vi "linear_system.vi"(4 "c(friction)":dbl, 5 "k(spring force)":dbl, 6 "delta_t":dbl, 7 "m(mass)":dbl, 8 "u_in(input force)":dbl, 9 "a_init":dbl, 10 "v_init":dbl, 11 "x_init":dbl) -> (1 "a_out":dbl, 2 "v_out":dbl, 3 "x_out":dbl)   [LabVIEW 2019]
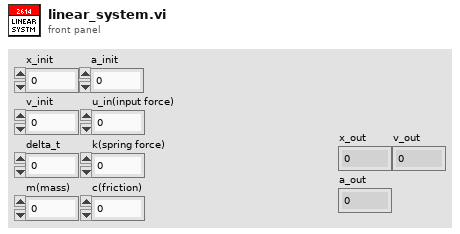
[diagram p1: front panel]
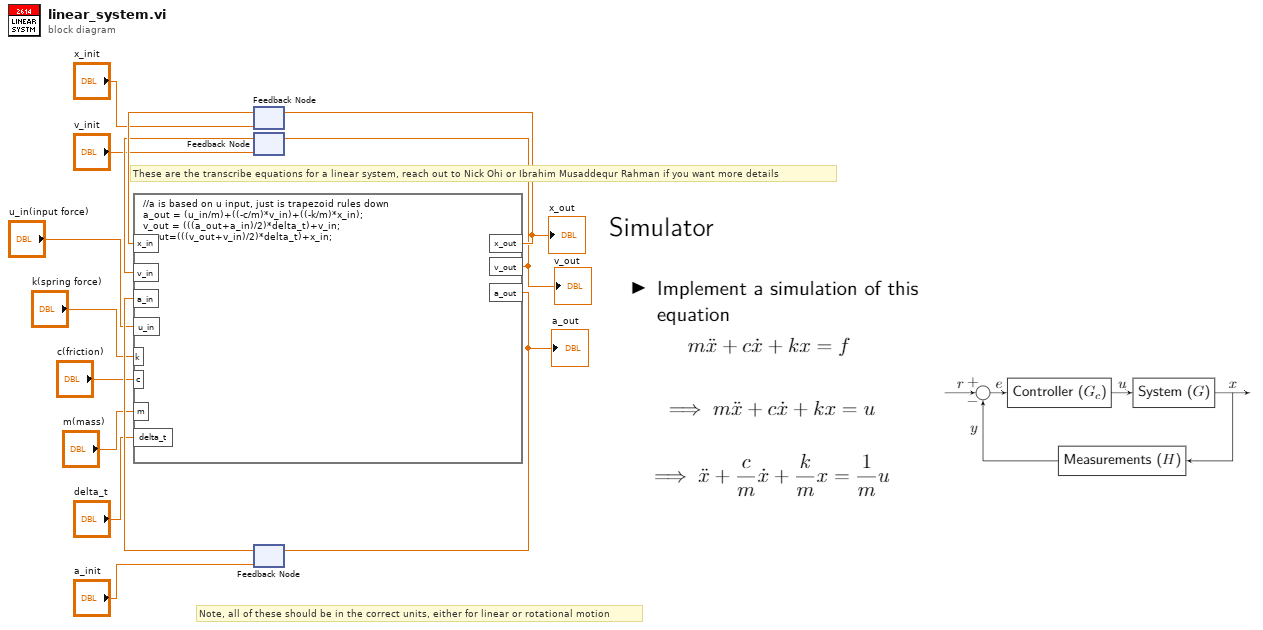
[diagram p0: block diagram]
diagram:
  # "These are the transcribe equations for a linear system, reach out to Nick Ohi or Ibrahim Musaddequr Rahman if you want more details"
  # "Note, all of these should be in the correct units, either for linear or rotational motion"
  n1 = feedback #1("x_init") -> (w14:dbl)
  n2 = feedback #2("v_init") -> (w10:dbl)
  n3 = feedback #3("a_init") -> (w7:dbl)
  n4 = formula code="//a is based on u input, just is trapezoid rules down\na_out = (u_in/m)+((-c/m)*v_in)+((-k/m)*x_in);\nv_out = (((a_out+a_in)/2)*delta_t)+v_in;\nx_out=(((v_out+v_in)/2)*delta_t)+x_in;"("x_in"=w14, "v_in"=w10, "a_in"=w7, "u_in"="u_in(input force)", "k"="k(spring force)", "c"="c(friction)", "m"="m(mass)", "delta_t"="delta_t") -> ("x_out"=w13:dbl, "v_out"=w11:dbl, "a_out"=w8:dbl)
  "x_out" <- w13
  "v_out" <- w11
  "a_out" <- w8
  n5 = feedback-in #1(w13) -> ()
  n6 = feedback-in #2(w11) -> ()
  n7 = feedback-in #3(w8) -> ()
